vi "Run.vi"(8 "error in (no error)":errorcluster, 11 "Car Position Simulator in":refnum<class "Car Position Simulator.lvclass">) -> (0 "error out":errorcluster, 3 "Car Position Simulator out":refnum<class "Car Position Simulator.lvclass">)   [LabVIEW 2016, in "CLD Exam - Car Wash.lvlib" / "Car Position Simulator.lvclass"]
doc: "--\nCopyright © 2017 Composed SystemsI All rights reserved.\n\nAuthor: Jon McBee <jon.mcbee@composed.io>\n\nThis library is provided \"AS IS\" ,WITHOUT WARRANTIES OR\nCONDITIONS OF ANY KIND, either express or implied.\n\nComposed Systems -- composed.io\n\nStream 0.0.1.1\nJon McBee - Composed Systems\nCopyright (c) 2017, Composed Systems"
uses:
  Car Position Simulator.lvclass
  D:/Repos/Stream/software/Mediator/Classes/Mediated Actor/Mediated Actor.lvclass
  Mediator/Classes/Message Interface/Message Interface.lvclass
  Car Position Simulator.lvclass/Car Position Simulator.ctl
  Car Wash Option Started Event/Car Wash Option Started.lvclass
  Car Position Changed Event/Car Position Changed.lvclass
  D:/Repos/Stream/software/Mediator/Classes/Message Interface/Message Interface.lvclass
  Mediator/Classes/Message Transport Queue/Message Transport Queue.lvclass
  Mediator/Classes/Mediated Actor/Mediated Actor.lvclass
panel:
  out "Active Option":string
  in  "Car Position Simulation":i32(slide) scale=0.0..4.0
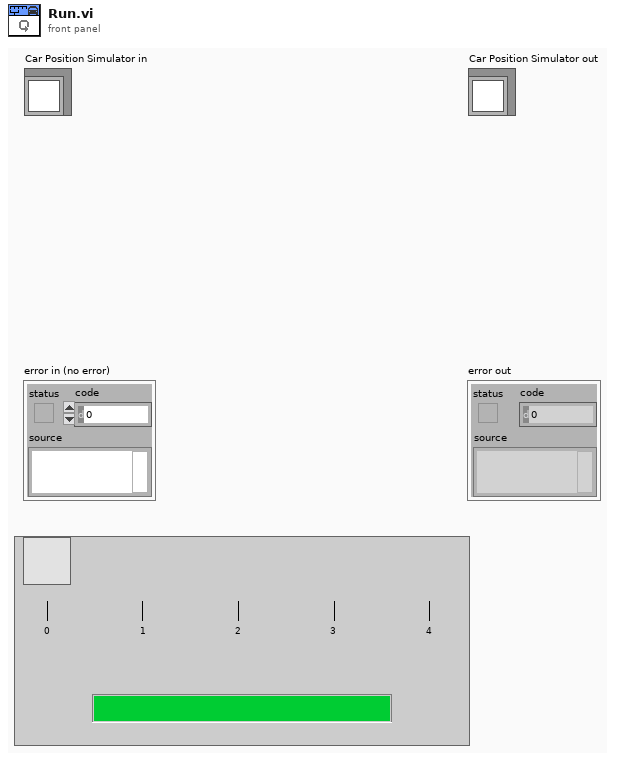
[diagram p1: front panel]
types:
  T1 = cluster{"System Exit":refnum<event-registration>, "To Self":refnum<event-registration>, "Vehicle Out of Position":refnum<event-registration>, "Car Wash Option Started":refnum<event-registration>, "Car Wash Finished":refnum<event-registration>, "Car Wash Started":refnum<event-registration>}
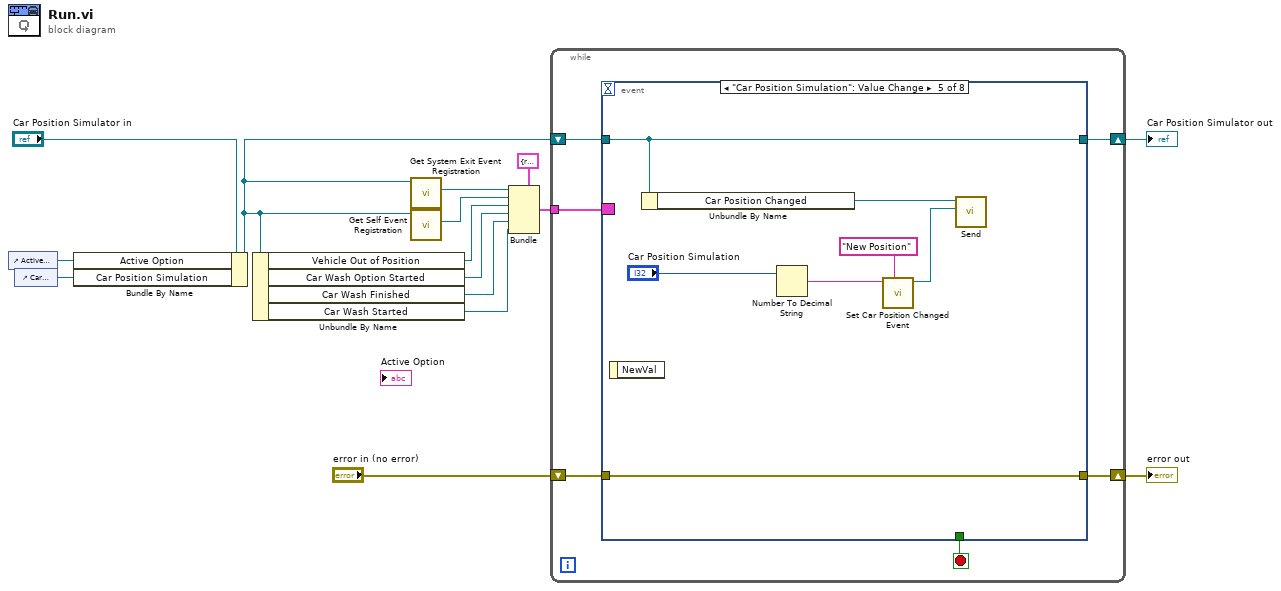
[diagram p0: block diagram]
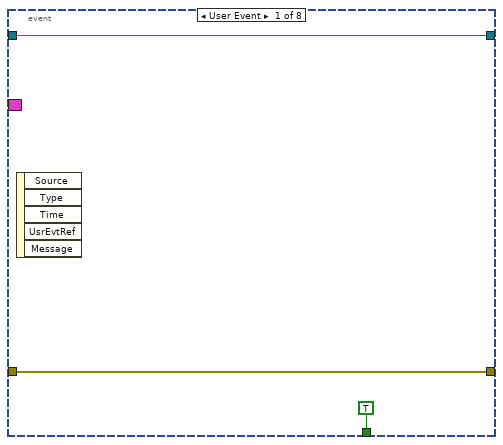
[diagram p2: hidden frame]
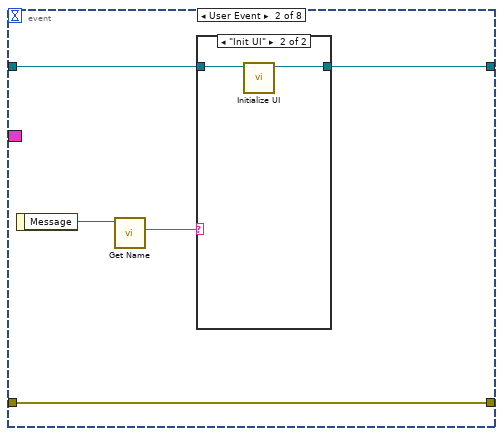
[diagram p3: hidden frame]
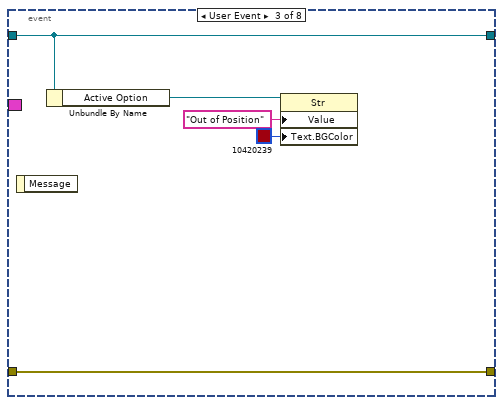
[diagram p5: hidden frame]
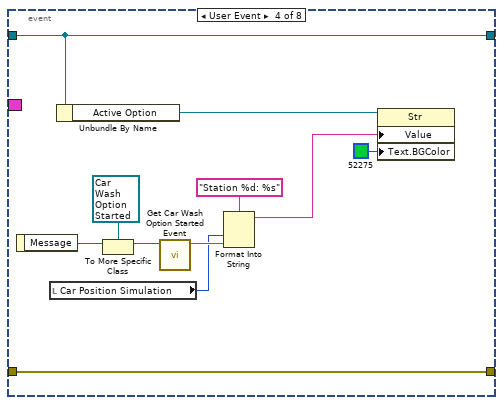
[diagram p6: hidden frame]
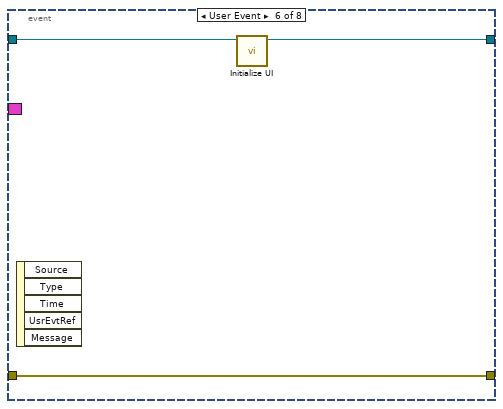
[diagram p7: hidden frame]
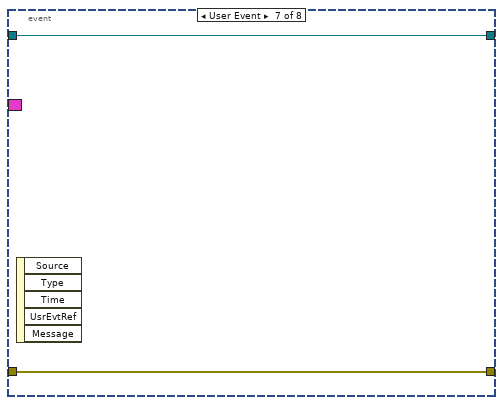
[diagram p8: hidden frame]
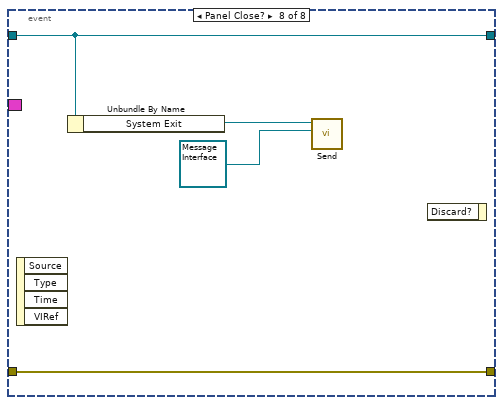
[diagram p9: hidden frame]
diagram:
  n1 = control-ref of="Active Option"() -> (w4:refnum<vi>)
  n2 = control-ref of="Car Position Simulation"() -> (w3:refnum<vi>)
  n3 = Bundle By Name(cluster="Car Position Simulator in", "Active Option"=w4, "Car Position Simulation"=w3) -> (w5:refnum<class "Car Position Simulator.lvclass">)
  n4 = Unbundle By Name(w5) -> ("Vehicle Out of Position"=w10:refnum<event-registration>, "Car Wash Option Started"=w9:refnum<event-registration>, "Car Wash Finished"=w2:refnum<event-registration>, "Car Wash Started"=w1:refnum<event-registration>)
  n5 = call "Get System Exit Event Registration.vi"("Mediated Actor in"=w5) -> ("System Exit Registration"=w12:refnum<event-registration>)  [unwired: 9 in, 1 out]
  n6 = call "Get Self Event Registration.vi"("Mediated Actor in"=w5) -> ("Event Registration Refnum"=w11:refnum<event-registration>)  [unwired: 9 in, 1 out]
  n7 = Bundle(cluster=T1 {"System Exit"=refnum, "To Self"=refnum, "Vehicle Out of Position"=refnum, "Car Wash Option Started"=refnum, "Car Wash Finished"=refnum, "Car Wash Started"=refnum} ("output cluster"), "System Exit"=w12, "To Self"=w11, "Vehicle Out of Position"=w10, "Car Wash Option Started"=w9, "Car Wash Finished"=w2, "Car Wash Started"=w1) -> (w7:T1)
  n8 = while {
    shift-right: [w20] -> w15
    shift-left: w5 -> [w21]
    shift-right: [w18] -> w13
    shift-left: "error in (no error)" -> [w19]
    tunnel: w7 -> [w17]
    stop <- w16 stop-if-true
    n9 = event shown="[4] \"Car Position Simulation\": Value Change" {
      selector: w17 -> [_ _ _ _ _ _ _ _]
      dyn-events: _ -> [_ _ _ _ _ _ _ _]
      timeout: _ -> [_ _ _ _ _ _ _ _]
      tunnel: w21 -> [w24 w27 w36 w46 w54 w57 w59 w63]
      tunnel: [w24 w26 w36 w46 w54 w56 w59 w63] -> w20
      tunnel: w19 -> [w23 w29 w37 w48 w55 w58 w60 w64]
      tunnel: [w23 w29 w37 w48 w55 w58 w60 w64] -> w18
      tunnel: [TRUE _ _ _ _ _ _ _] -> w16
      event User Event {
        n10 = event-data() -> ()  [unwired: 1 in, 5 out]
      }
      event User Event {
        n11 = event-data() -> ("Message"=w28:refnum<class "Message Interface.lvclass">)  [unwired: 1 in]
        n12 = call "Get Name.vi"("Message Interface in"=w28) -> ("Name"=w25:string)  [unwired: 8 in, 2 out]
        n13 = case shown="\"Init UI\"" w25 {
          tunnel: w27 -> [w30 w32]
          tunnel: [w30 w31] -> w26
          frame Default {
          }
          frame "Init UI" {
            n14 = call "Initialize UI.vi"("Car Position Simulator in"=w32) -> ("Car Position Simulator out"=w31:refnum<class "Car Position Simulator.lvclass">)  [unwired: 10 in]
          }
        }
      }
      event User Event {
        n15 = event-data() -> ()  [unwired: 1 in, 1 out]
        n16 = Unbundle By Name(w36) -> ("Active Option"=w35:refnum<vi>)
        n17 = property class="Str"(reference=w35, "Value"="Out of Position", "Text.BGColor"=u32 10420239) -> ()  [unwired: 1 in, 2 out]
      }
      event User Event {
        n18 = event-data() -> ("Message"=w44:refnum<class "Message Interface.lvclass">)  [unwired: 1 in]
        n19 = local read "Car Position Simulation"() -> (w39:i32)
        n20 = Unbundle By Name(w46) -> ("Active Option"=w45:refnum<vi>)
        n21 = To More Specific Class(target class=refnum<class "Car Wash Option Started.lvclass"> refnum ("Car Wash Option Started.lvclass"), reference=w44) -> (specific class reference=w42:refnum<class "Car Wash Option Started.lvclass">)  [unwired: 1 in, 1 out]
        n22 = call "Get Car Wash Option Started Event.vi"("Car Wash Option Started in"=w42) -> ("Option"=w40:string)  [unwired: 9 in, 1 out]
        n23 = Format Into String(format string="Station %d: %s" ("Value"), w39, w40) -> (resulting string=w38:string)  [unwired: 2 in, 1 out]
        n24 = property class="Str"(reference=w45, "Value"=w38, "Text.BGColor"=u32 52275) -> ()  [unwired: 1 in, 2 out]
      }
      event "Car Position Simulation": Value Change {
        n25 = event-data() -> ()  [unwired: 1 in, 1 out]
        n26 = Unbundle By Name(w54) -> ("Car Position Changed"=w53:refnum<class "Message Transport Queue.lvclass">)
        n27 = Number To Decimal String(number="Car Position Simulation") -> (decimal integer string=w49:string)  [unwired: 1 in]
        n28 = call "Set Car Position Changed Event.vi"("Name"="New Position", "Station"=w49) -> ("Car Position Changed out"=w52:refnum<class "Car Position Changed.lvclass">)  [unwired: 9 in]
        n29 = call-dynamic "Send.vi"("Message"=w52, "Message Transport Queue in"=w53) -> ()  [unwired: 7 in, 3 out]
      }
      event User Event {
        n30 = event-data() -> ()  [unwired: 1 in, 5 out]
        n31 = call "Initialize UI.vi"("Car Position Simulator in"=w57) -> ("Car Position Simulator out"=w56:refnum<class "Car Position Simulator.lvclass">)  [unwired: 10 in]
      }
      event User Event {
        n32 = event-data() -> ()  [unwired: 1 in, 5 out]
      }
      event Panel Close? {
        n33 = event-data() -> ()  [unwired: 1 in, 4 out]
        n34 = Unbundle By Name(w63) -> ("System Exit"=w62:refnum<class "Message Transport Queue.lvclass">)
        n35 = call-dynamic "Send.vi"("Message"=refnum<class "Message Interface.lvclass"> refnum, "Message Transport Queue in"=w62) -> ()  [unwired: 7 in, 3 out]
        n36 = event-data() -> ()  [unwired: 2 in, 1 out]
      }
    }
  }
  "error out" <- w13
  "Car Position Simulator out" <- w15
